vi "Interface_Test.vi"() -> ()   [LabVIEW 2014]
uses:
  <vilib>/Utility/miscctls.llb/LVRectTypeDef.ctl
panel:
  out "result string":string
  out "path":path
  out "x-y*floor(x/y)":i32
  in  "stop":bool
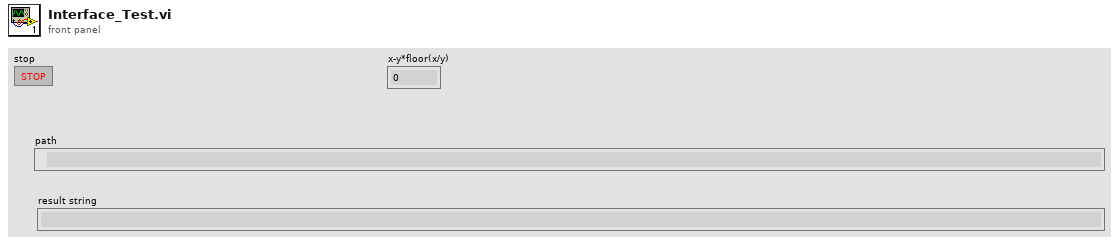
[diagram p1: front panel]
types:
  T1 = typedef "LVRectTypeDef.ctl" = cluster{"Left":i16, "Top":i16, "Right":i16, "Bottom":i16}
  T2 = enum32{"Invalid", "Standard", "Closed", "Hidden", "Minimized", "Maximized"}
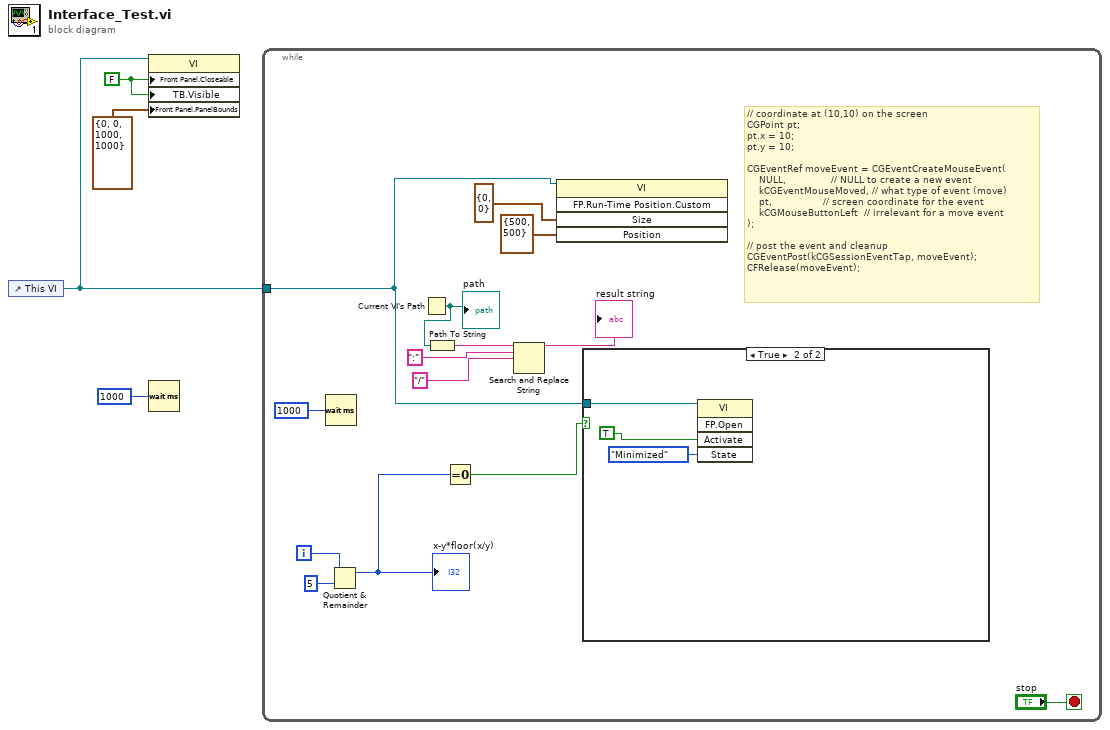
[diagram p0: block diagram]
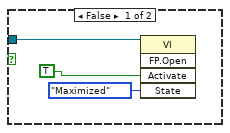
[diagram p2: hidden frame]
diagram:
  w4 = FALSE ("Front Panel Window:Is Frontmost")
  n1 = control-ref of="This VI"() -> (w2:refnum<vi>)
  n2 = property class="VI"(reference=w2, "Front Panel.Closeable"=w4, "TB.Visible"=w4, "Front Panel.PanelBounds"=T1 {"Left"=0, "Top"=0, "Right"=1000, "Bottom"=1000} ("Front Panel Window:Panel Bounds")) -> ()  [unwired: 1 in, 2 out]
  n3 = Wait (ms)(milliseconds to wait=u32 1000) -> ()  [unwired: 1 out]
  n4 = while {
    tunnel: w2 -> [w5]
    i -> [w17]
    stop <- "stop" stop-if-true
    # "// coordinate at (10,10) on the screen\nCGPoint pt;\npt.x = 10;\npt.y = 10;\n\nCGEventRef moveEvent = CGEventCreateMouseEvent(\n    NULL,               // NULL to create a new event\n    kCGEventMouseMoved, // what type of event (move)\n    pt,                 // screen coordinate for the event\n    kCGMouseButtonLeft  // irrelevant for a move event\n);\n\n// post the event and cleanup\nCGEventPost(kCGSessionEventTap, moveEvent);\nCFRelease(moveEvent);"
    n5 = Wait (ms)(milliseconds to wait=u32 1000) -> ()  [unwired: 1 out]
    n6 = Quotient & Remainder(x=w17, y=5) -> (x-y*floor(x/y)=w13:i32)  [unwired: 1 out]
    "x-y*floor(x/y)" <- w13
    n7 = Current VI's Path() -> (path=w10:path)
    "path" <- w10
    n8 = Path To String(path=w10) -> (string=w9:string)
    n9 = Equal To 0?(x=w13) -> (x = 0?=w14:bool)
    n10 = Search and Replace String(input string=w9, search string=":", replace string="/" ("replace string (\"\")")) -> (result string=→"result string":string)  [unwired: 5 in, 3 out]
    n11 = invoke class="VI" method="FP.Run-Time Position.Custom"(reference=w5, "Size"=cluster{"Top":i16, "Left":i16} {"Top"=0, "Left"=0} ("Position"), "Position"=cluster{"Height":i16, "Width":i16} {"Height"=500, "Width"=500} ("Size")) -> ()  [unwired: 2 in, 5 out]
    n12 = case shown="True" w14 {
      tunnel: w5 -> [w19 w22]
      frame False {
        n13 = invoke class="VI" method="FP.Open"(reference=w19, "Activate"=TRUE, "State"=T2."Maximized") -> ()  [unwired: 2 in, 5 out]
      }
      frame True {
        n14 = invoke class="VI" method="FP.Open"(reference=w22, "Activate"=TRUE, "State"=T2."Minimized") -> ()  [unwired: 2 in, 5 out]
      }
    }
  }
